vi "TestEncodeArrayFloat32(Auto-Concatenating).vi"(8 "error in (no error)":errorcluster, 11 "Single Array":sgl[](array[numeric])) -> (0 "error out":errorcluster, 3 "MessagePack":u8[](array[numeric]) format="%.0x")   [LabVIEW 2015, in "MsgPack.lvlib"]
uses:
  MsgPack.lvlib
  EncodeTypes/encodeFloat32.vi
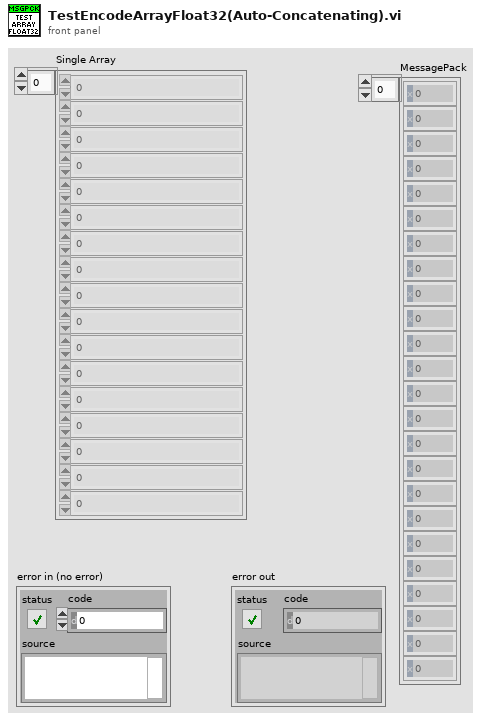
[diagram p1: front panel]
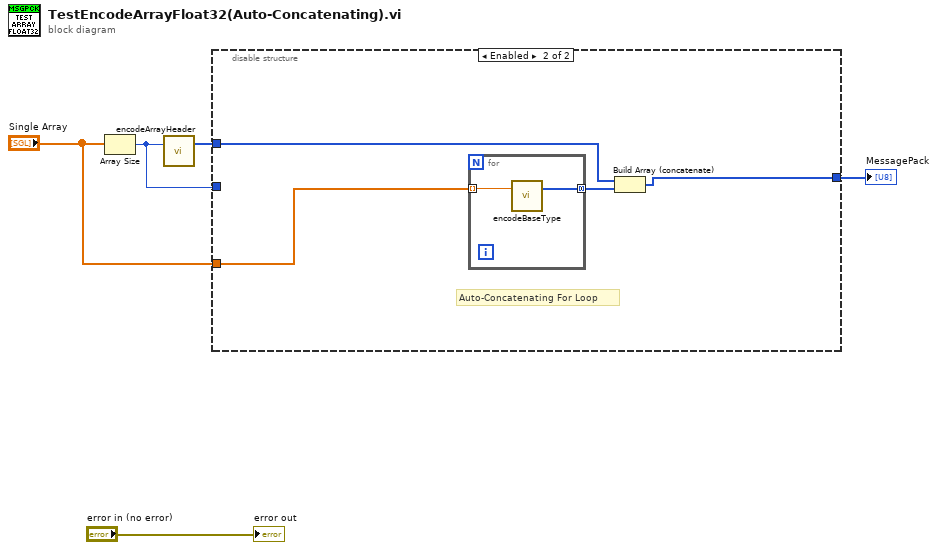
[diagram p0: block diagram]
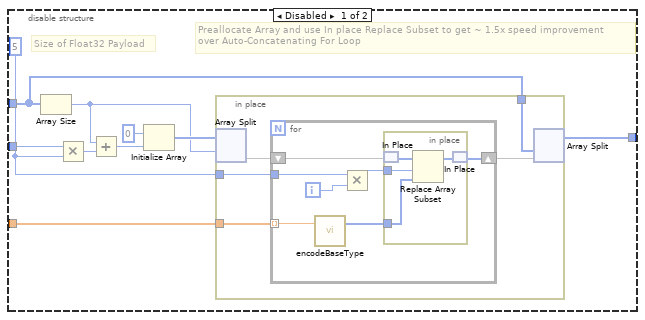
[diagram p2: hidden frame]
diagram:
  n1 = Array Size(array="Single Array") -> (size(s)=w4:i32)
  n2 = call "encodeArrayHeader.vi"("Number of Elements"=w4) -> ("array header"=w2:u8[])  [unwired: 2 in]
  n3 = disable-structure shown="Enabled" {
    disable-tunnel: [w9 w32] -> w5
    disable-tunnel: w4 -> [w8 _]
    disable-tunnel: "Single Array" -> [w7 w33]
    disable-tunnel: w2 -> [w6 w34]
    frame Disabled {
      w10 = 5 ("y")
      # "Preallocate Array and use In place Replace Subset to get ~ 1.5x speed improvement\nover Auto-Concatenating For Loop"
      # "Size of Float32 Payload"
      n4 = Array Size(array=w6) -> (size(s)=w11:i32)
      n5 = Multiply(x=w8, y=w10) -> (x*y=w14:i32)
      n6 = Add(x=w11, y=w14) -> (x+y=w13:i32)
      n7 = Initialize Array(u8 0, w13) -> (w12:u8[])
      n8 = in-place {
        in-place-border: w6 -> [w20]
        in-place-border: w7 -> [w19]
        in-place-border: w10 -> [w16]
        n9 = in-place-split #1(w12, w11) -> (w18:u8[])  [unwired: 1 out]
        n10 = for {
          tunnel: w19 -> [w22] mode=indexing
          shift-right: [w26] -> w17
          shift-left: w18 -> [w27]
          tunnel: w16 -> [w24]
          i -> [w25]
          n11 = call-poly "encodeBaseType.vi"("Float32"=w22) -> ("MessagePack"=w21:u8[])  [unwired: 2 in]
          n12 = Multiply(x=w24, y=w25) -> (x*y=w23:i32)
          n13 = in-place {
            in-place-border: w21 -> [w29]
            in-place-border: w23 -> [w28]
            n14 = in-place-match #2(w27) -> (w31:u8[])
            n15 = Replace Array Subset(array=w31, new element=w29, index=w28) -> (w30:u8[])
            n16 = in-place-match #2(w30) -> (w26:u8[])
          }
        }
        n17 = in-place-split #1(w20, w17) -> (w9:u8[])  [unwired: 1 out]
      }
    }
    frame Enabled {
      # "Auto-Concatenating For Loop"
      n18 = for {
        tunnel: w33 -> [w37] mode=indexing
        tunnel: [w36] -> w35 mode=concatenating
        n19 = call-poly "encodeBaseType.vi"("Float32"=w37) -> ("MessagePack"=w36:u8[])  [unwired: 2 in]
      }
      n20 = Build Array (concatenate)(w34, w35) -> (w32:u8[])
    }
  }
  "MessagePack" <- w5
  "error out" <- "error in (no error)"
